vi "Write Message Stream.vi"(10 "Message Stream":refnum<class "Message Stream.lvclass">, 11 "Chat Window in":refnum<class "Chat Window.lvclass">) -> (3 "Chat Window out":refnum<class "Chat Window.lvclass">)   [LabVIEW 2020, in "Chat Window.lvlib" / "Chat Window.lvclass"]
doc: "Use this VI to specify the type of message stream to be used by this actor's nested endpoint."
uses:
  Chat Window.lvclass
  Nested Endpoint Actors/Abstract Classes/Message Stream/Message Stream.lvclass
  Chat Window.lvclass/Chat Window.ctl
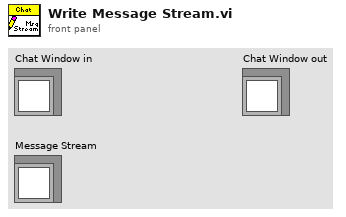
[diagram p1: front panel]
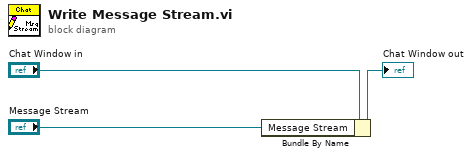
[diagram p0: block diagram]
diagram:
  n1 = Bundle By Name(cluster="Chat Window in", "Message Stream"="Message Stream") -> (→"Chat Window out":refnum<class "Chat Window.lvclass">)
